vi "getWaypoints.vi"(8 "Error In":errorcluster, 11 "StationKeeping in":refnum<class "StationKeeping.lvclass">) -> (0 "Error Out":errorcluster, 2 "Waypoint Array":refnum<class "Waypoint.lvclass">[](array[class]), 3 "StationKeeping out":refnum<class "StationKeeping.lvclass">)   [LabVIEW 2013, in "StationKeeping.lvclass"]
doc: "Generate and get the critical points for this mission. In this case, it creates a waypoint between the first and second defined points if we still need to stay in the box, and clears the array if not."
uses:
  StationKeeping.lvclass
  Waypoint/Waypoint.lvclass
  GenericMission/GenericMission.lvclass
  StationKeeping.lvclass/StationKeeping.ctl
panel:
  in  "y":timestamp
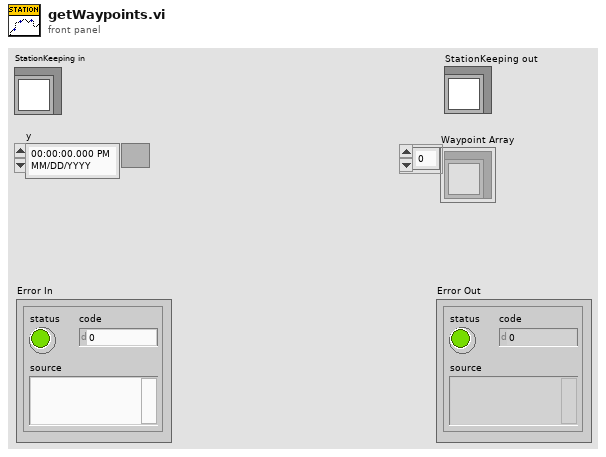
[diagram p1: front panel]
types:
  T1 = typedef "UTM Location.ctl" = cluster{"UTM Zone":dbl, "Hemisphere":enum16{"North", "South"}, "East":dbl, "North":dbl}
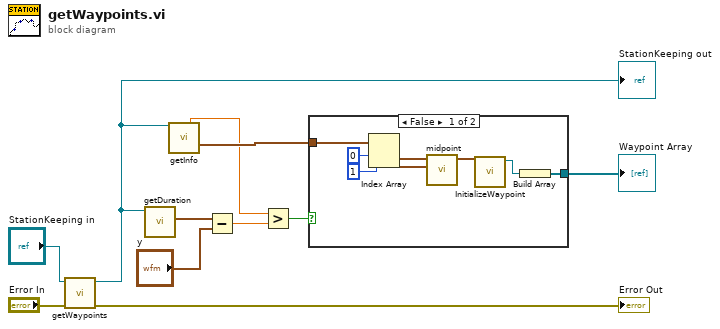
[diagram p0: block diagram]
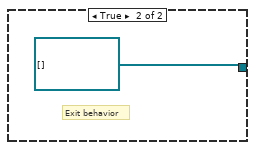
[diagram p2: hidden frame]
diagram:
  n1 = call-parent "getWaypoints.vi"("Error In"="Error In", "GenericMission in"="StationKeeping in") -> ("Error Out"=→"Error Out":errorcluster, "GenericMission out"=w4:refnum<class "StationKeeping.lvclass">)  [unwired: 7 in, 1 out]
  "StationKeeping out" <- w4
  n2 = call "getDuration.vi"("StationKeeping in"=w4) -> ("Duration"=w3:timestamp)  [unwired: 8 in, 2 out]
  n3 = call-dynamic "getInfo.vi"("GenericMission in"=w4) -> ("Duration (s)"=w1:dbl, "Points of Interest"=w6:T1[])  [unwired: 6 in, 7 out]
  n4 = Subtract(x=w3, y="y") -> (x-y=w2:dbl)
  n5 = Greater?(x=w1, y=w2) -> (0:w8:bool)
  n6 = case shown="False" w8 {
    tunnel: w6 -> [w13 _]
    tunnel: [w12 refnum<class "Waypoint.lvclass">[] []] -> w7
    frame False {
      n7 = Index Array(array=w13, index #1=0 ("index"), index #2=1 ("index")) -> (element #1=w17:T1, element #2=w16:T1)
      n8 = call "midpoint.vi"("UTM Location 2"=w16, "UTM Location"=w17) -> ("UTM Location 3"=w14:T1)  [unwired: 8 in, 1 out]
      n9 = call "InitializeWaypoint.vi"("Coords"=w14) -> ("Waypoint Out"=w15:refnum<class "Waypoint.lvclass">)  [unwired: 10 in]
      n10 = Build Array(w15) -> (w12:refnum<class "Waypoint.lvclass">[])
    }
    frame True {
      # "Exit behavior"
    }
  }
  "Waypoint Array" <- w7
